vi "runTestScenario.vi"(0 "Constant Analog Output Voltage Test  in":refnum<class "Current Linear Test.lvclass">, 5 "ILC":refnum<class "ILC.lvclass">, 11 "error in (no error)":errorcluster) -> (4 "Constant Analog Output Voltage Test  out":refnum<class "Current Linear Test.lvclass">, 6 "ILC 2":refnum<class "ILC.lvclass">, 8 "TestExecution":T2, 10 "Result":T1, 15 "error out":errorcluster)   [LabVIEW 2016, in "Current Linear Test.lvclass"]
uses:
  Current Linear Test.lvclass
  Typedefs/TestExecution.ctl
  Typedefs/PassFailTest.ctl
  Common_ILC/ILC/ILC.lvclass
  Typedefs/WriteDataFileInput.ctl
  Typedefs/TestScenarioTypes.ctl
  Typedefs/WriteLogMessageInput.ctl
  Current Linear Test.lvclass/Current Linear Test.ctl
  Model/TestLog/ITestLog/ITestLog.lvclass
  Model/ConfigureILCStrategy/IConfigureILCStrategy/IConfigureILCStrategy.lvclass
  Typedefs/ILCBTTypedefs.lvlib
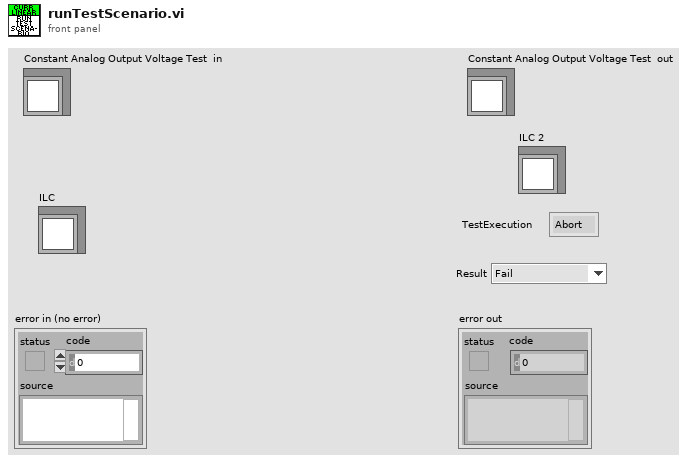
[diagram p1: front panel]
types:
  T1 = typedef "ILCBTTypedefs.lvlib/PassFailTest.ctl" = enum16{"Fail", "Pass", "NA"}
  T2 = typedef "ILCBTTypedefs.lvlib/TestExecution.ctl" = enum16{"Abort", "Continue"}
  T3 = typedef "ILCBTTypedefs.lvlib/WriteLogMessageInput.ctl" = cluster{"Test Scenario":T4, "Description":string, "Actual Value":string, "Data File":string, "Result":T1}
  T4 = typedef "ILCBTTypedefs.lvlib/TestScenarioTypes.ctl" = enum16{"+3.3VD", "+5.1V", "+24V", "RELVALV1", "RELVALV2", "Verify DAC_A = -1.00A", "Verify DAC_A = -0.75A", "Verify DAC_A = -0.50A", "Verify DAC_A = -0.25A", "Verify DAC_A = 0.00A", "Verify DAC_A = 0.25A", "Verify DAC_A = 0.50A", "Verify DAC_A = 0.75A", "Verify DAC_A = 1.00A", "Verify DAC_B = -1.00A", "Verify DAC_B = -0.75A", "Verify DAC_B = -0.50A", "Verify DAC_B = -0.25A", "Verify DAC_B = 0.00A", "Verify DAC_B = 0.25A", "Verify DAC_B = 0.50A", "Verify DAC_B = 0.75A", "Verify DAC_B = 1.00A", "Set DAC_A = -1.00A", "Set DAC_A = -0.75A", "Set DAC_A = -0.50A", "Set DAC_A = -0.25A", "Set DAC_A = 0.00A", "Set DAC_A = 0.25A", "Set DAC_A = 0.50A", "Set DAC_A = 0.75A", "Set DAC_A = 1.00A", "Set DAC_B = -1.00A", "Set DAC_B = -0.75A", "Set DAC_B = -0.50A", "Set DAC_B = -0.25A", "Set DAC_B = 0.00A", "Set DAC_B = 0.25A", "Set DAC_B = 0.50A", "Set DAC_B = 0.75A", "Set DAC_B = 1.00A", "Set MTR_PWR = On", "Set MTR_PWR = Off", "Set OUTPUT = On", "Set OUTPUT = Off", "Verify OUTPUT = On", "Verify OUTPUT = Off", "Verify POWER = Ok", "Verify POWER = Fail", "Verify AMP1 = Ok", "Verify AMP1 = Fail", "Verify AMP2 = Ok", "Verify AMP2 = Fail", "P1 0%", "P1 25%", "P1 50%", "P1 75%", "P1 100%", "P2 0%", "P2 25%", "P2 50%", "P2 75%", "P2 100%", "P3 0%", "P3 25%", "P3 50%", "P3 75%", "P3 100%", "P4 0%", "P4 25%", "P4 50%", "P4 75%", "P4 100%", "DCA 1 Linearity", "DCA 2 Linearity"}
  T5 = typedef "ILCBTTypedefs.lvlib/WriteDataFileInput.ctl" = cluster{"Test Scenario":T4, "File Name":string, "Output":string[]}
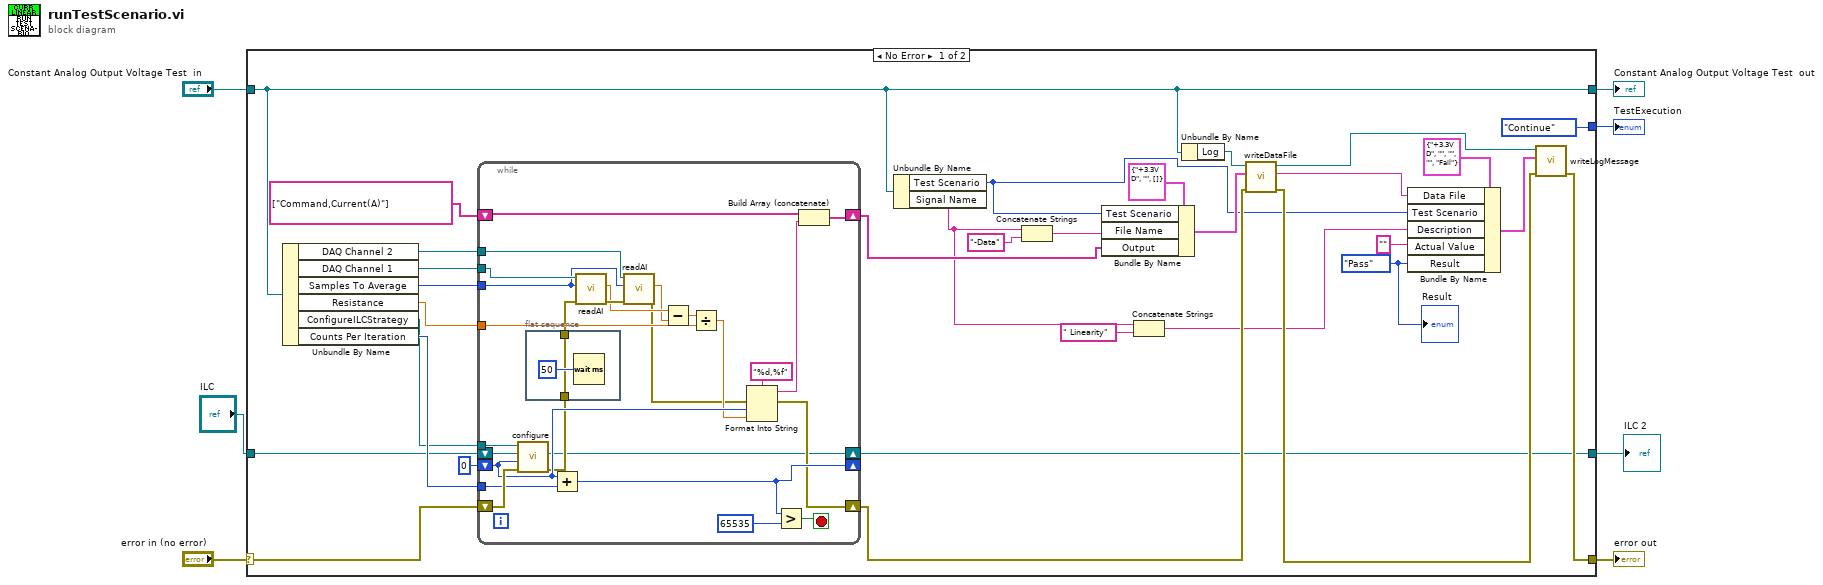
[diagram p0: block diagram]
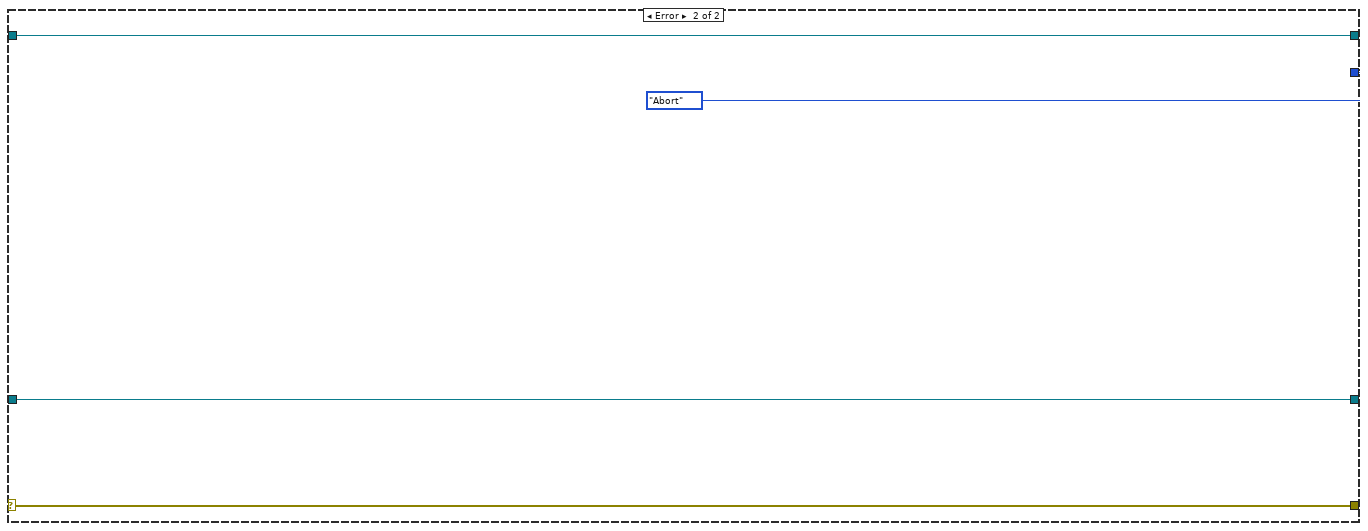
[diagram p2: hidden frame]
diagram:
  n1 = case shown="No Error" "error in (no error)" {
    selector: "error in (no error)" -> [w30 w71]
    tunnel: [w11 w71] -> w6
    tunnel: [TestExecution."Continue" ("TestExecution") TestExecution."Abort" ("TestExecution")] -> w5
    tunnel: "Constant Analog Output Voltage Test  in" -> [w9 w69]
    tunnel: [w9 w69] -> w3
    tunnel: "ILC" -> [w35 w68]
    tunnel: [w8 w68] -> w1
    frame No Error {
      w10 = PassFailTest."Pass" ("Result")
      n2 = Unbundle By Name(w9) -> ("DAQ Channel 2"=w32:refnum<k21>, "DAQ Channel 1"=w33:refnum<k21>, "Samples To Average"=w34:i32, "Resistance"=w31:dbl, "ConfigureILCStrategy"=w36:refnum<class "IConfigureILCStrategy.lvclass">, "Counts Per Iteration"=w37:i32)
      n3 = while {
        tunnel: w37 -> [w62]
        shift-right: [w49] -> _
        shift-left: u32 0 -> [w52]
        tunnel: w36 -> [w65]
        shift-right: [w44] -> w22
        shift-left: w30 -> [w63]
        tunnel: w34 -> [w58]
        tunnel: w33 -> [w60]
        tunnel: w32 -> [w59]
        tunnel: w31 -> [w54]
        shift-right: [w41] -> w26
        shift-left: string[] ["Command,Current(A)"] -> [w43]
        shift-right: [w40] -> w8
        shift-left: w35 -> [w64]
        stop <- w47 stop-if-true
        n4 = call-dynamic "configure.vi"("error in (no error)"=w63, "Value"=w52, "ILC"=w64, "IConfigureILCStrategy in"=w65) -> ("error out"=w46:errorcluster, "ILC 2"=w40:refnum<class "ILC.lvclass">)  [unwired: 5 in, 1 out]
        n5 = flat-sequence {
          tunnel: w46 -> [w66]
          tunnel: [w66] -> w45
          frame #0 {
            n6 = Wait (ms)(milliseconds to wait=u32 50) -> ()  [unwired: 1 out]
          }
        }
        n7 = Add(x=w52, y=w62) -> (x+y=w49:u32)
        n8 = call "readAI.vi"("error in (no error)"=w45, "Samples To Read"=w58, "DAQ Channel To Read"=w60) -> ("error out"=w61:errorcluster, "Average"=w57:dbl)  [unwired: 6 in, 1 out]
        n9 = call "readAI.vi"("error in (no error)"=w61, "Samples To Read"=w58, "DAQ Channel To Read"=w59) -> ("error out"=w50:errorcluster, "Average"=w56:dbl)  [unwired: 6 in, 1 out]
        n10 = Subtract(x=w57, y=w56) -> (x-y=w55:dbl)
        n11 = Divide(x=w55, y=w54) -> (x/y=w51:dbl)
        n12 = Format Into String(format string="%d,%f", error in=w50, w52, w51) -> (resulting string=w42:string, error out=w44:errorcluster)  [unwired: 1 in]
        n13 = Greater?(x=w49, y=u32 65535) -> (0:w47:bool)
        n14 = Build Array (concatenate)(w43, w42) -> (w41:string[])
      }
      n15 = Unbundle By Name(w9) -> ("Test Scenario"=w12:T4, "Signal Name"=w15:string)
      n16 = Concatenate Strings(w15, "-Data" ("string")) -> (w28:string)
      n17 = Bundle By Name(cluster=T5 {"Test Scenario"=enum."+3.3VD", "File Name"="", "Output"=[]} ("WriteDataFileInput"), "Test Scenario"=w12, "File Name"=w28, "Output"=w26) -> (w23:T5)
      n18 = Concatenate Strings(w15, " Linearity" ("string")) -> (w13:string)
      n19 = Unbundle By Name(w9) -> ("Log"=w24:refnum<class "ITestLog.lvclass">)
      n20 = call-dynamic "writeDataFile.vi"("error in (no error)"=w22, "WriteDataFileInput"=w23, "ITestLog in"=w24) -> ("error out"=w17:errorcluster, "Relative Path"=w18:string, "ITestLog out"=w21:refnum<class "ITestLog.lvclass">)  [unwired: 6 in]
      n21 = Bundle By Name(cluster=T3 {"Test Scenario"=enum."+3.3VD", "Description"="", "Actual Value"="", "Data File"="", "Result"=enum."Fail"} ("WriteLogMessageInput"), "Data File"=w18, "Test Scenario"=w12, "Description"=w13, "Actual Value"="", "Result"=w10) -> (w19:T3)
      n22 = call-dynamic "writeLogMessage.vi"("error in (no error)"=w17, "WriteLogMessageInput"=w19, "ITestLog in"=w21) -> ("error out"=w11:errorcluster)  [unwired: 7 in, 1 out]
      "Result" <- w10
    }
    frame Error {
    }
  }
  "Constant Analog Output Voltage Test  out" <- w3
  "error out" <- w6
  "TestExecution" <- w5
  "ILC 2" <- w1
